vi "TEST.vi"() -> ()   [LabVIEW 2014]
uses:
  <vilib>/Instr/_visa.llb/VISA Configure Serial Port (Instr).vi
panel:
  in  "Delay":u32=1000
  in  "Network":bool
  out "Axis":string="L127M127R127"
  in  "포트":u16=50
  in  "IP":string="127.0.0.1"
  out "불리언":bool=TRUE
  out "Write":string="L127,M127,R127,;\r"
  in  "Motor R":u32(slide)=128 scale=0.0..255.0
  in  "Motor M":u32(slide)=128 scale=0.0..255.0
  in  "Motor L":u32(slide)=128 scale=0.0..255.0
  in  "정지 버튼":bool
  in  "RUN":bool
  out "WORK":i32=34
  in  "VISA resource name":refnum<visa-resource-name>="COM3"
  in  "Serial Settings":T1={"baud rate"=9600, "data bits"=8, "parity"=enum."None", "stop bits"=10, "flow control"=0} {"flow control" items=["None"=0, "XON/XOFF"=1, "RTS/CTS"=2, "DTR/DSR"=4]; "stop bits" items=["1.0"=10, "1.5"=15, "2.0"=20]; "data bits" min=5 max=8 step=1; "baud rate" items=["75"=75, "110"=110, "134"=134, "150"=150, "300"=300, "600"=600, "1200"=1200, "1800"=1800, "2400"=2400, "4800"=4800, "7200"=7200, "9600"=9600, "14400"=14400, "19200"=19200, "28800"=28800, "38400"=38400, "56000"=56000, "57600"=57600, "115200"=115200, "128000"=128000, "230400"=230400]}
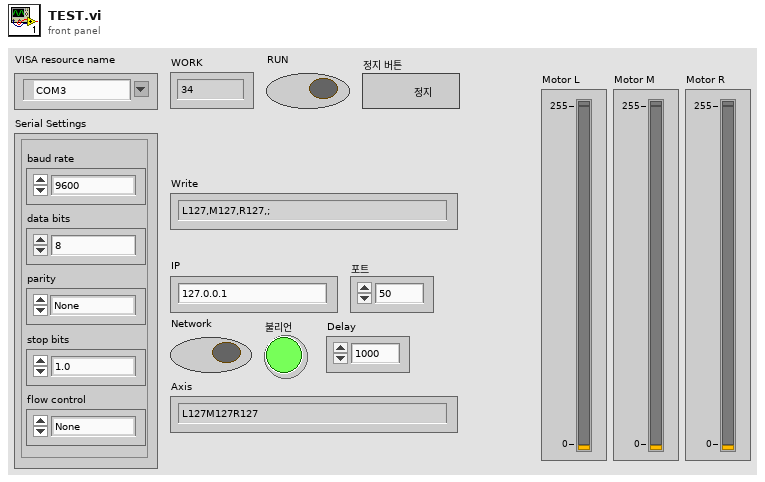
[diagram p1: front panel]
types:
  T1 = cluster{"baud rate":u32, "data bits":u16, "parity":enum16{"None", "Odd", "Even", "Mark", "Space"}, "stop bits":u16, "flow control":u16}
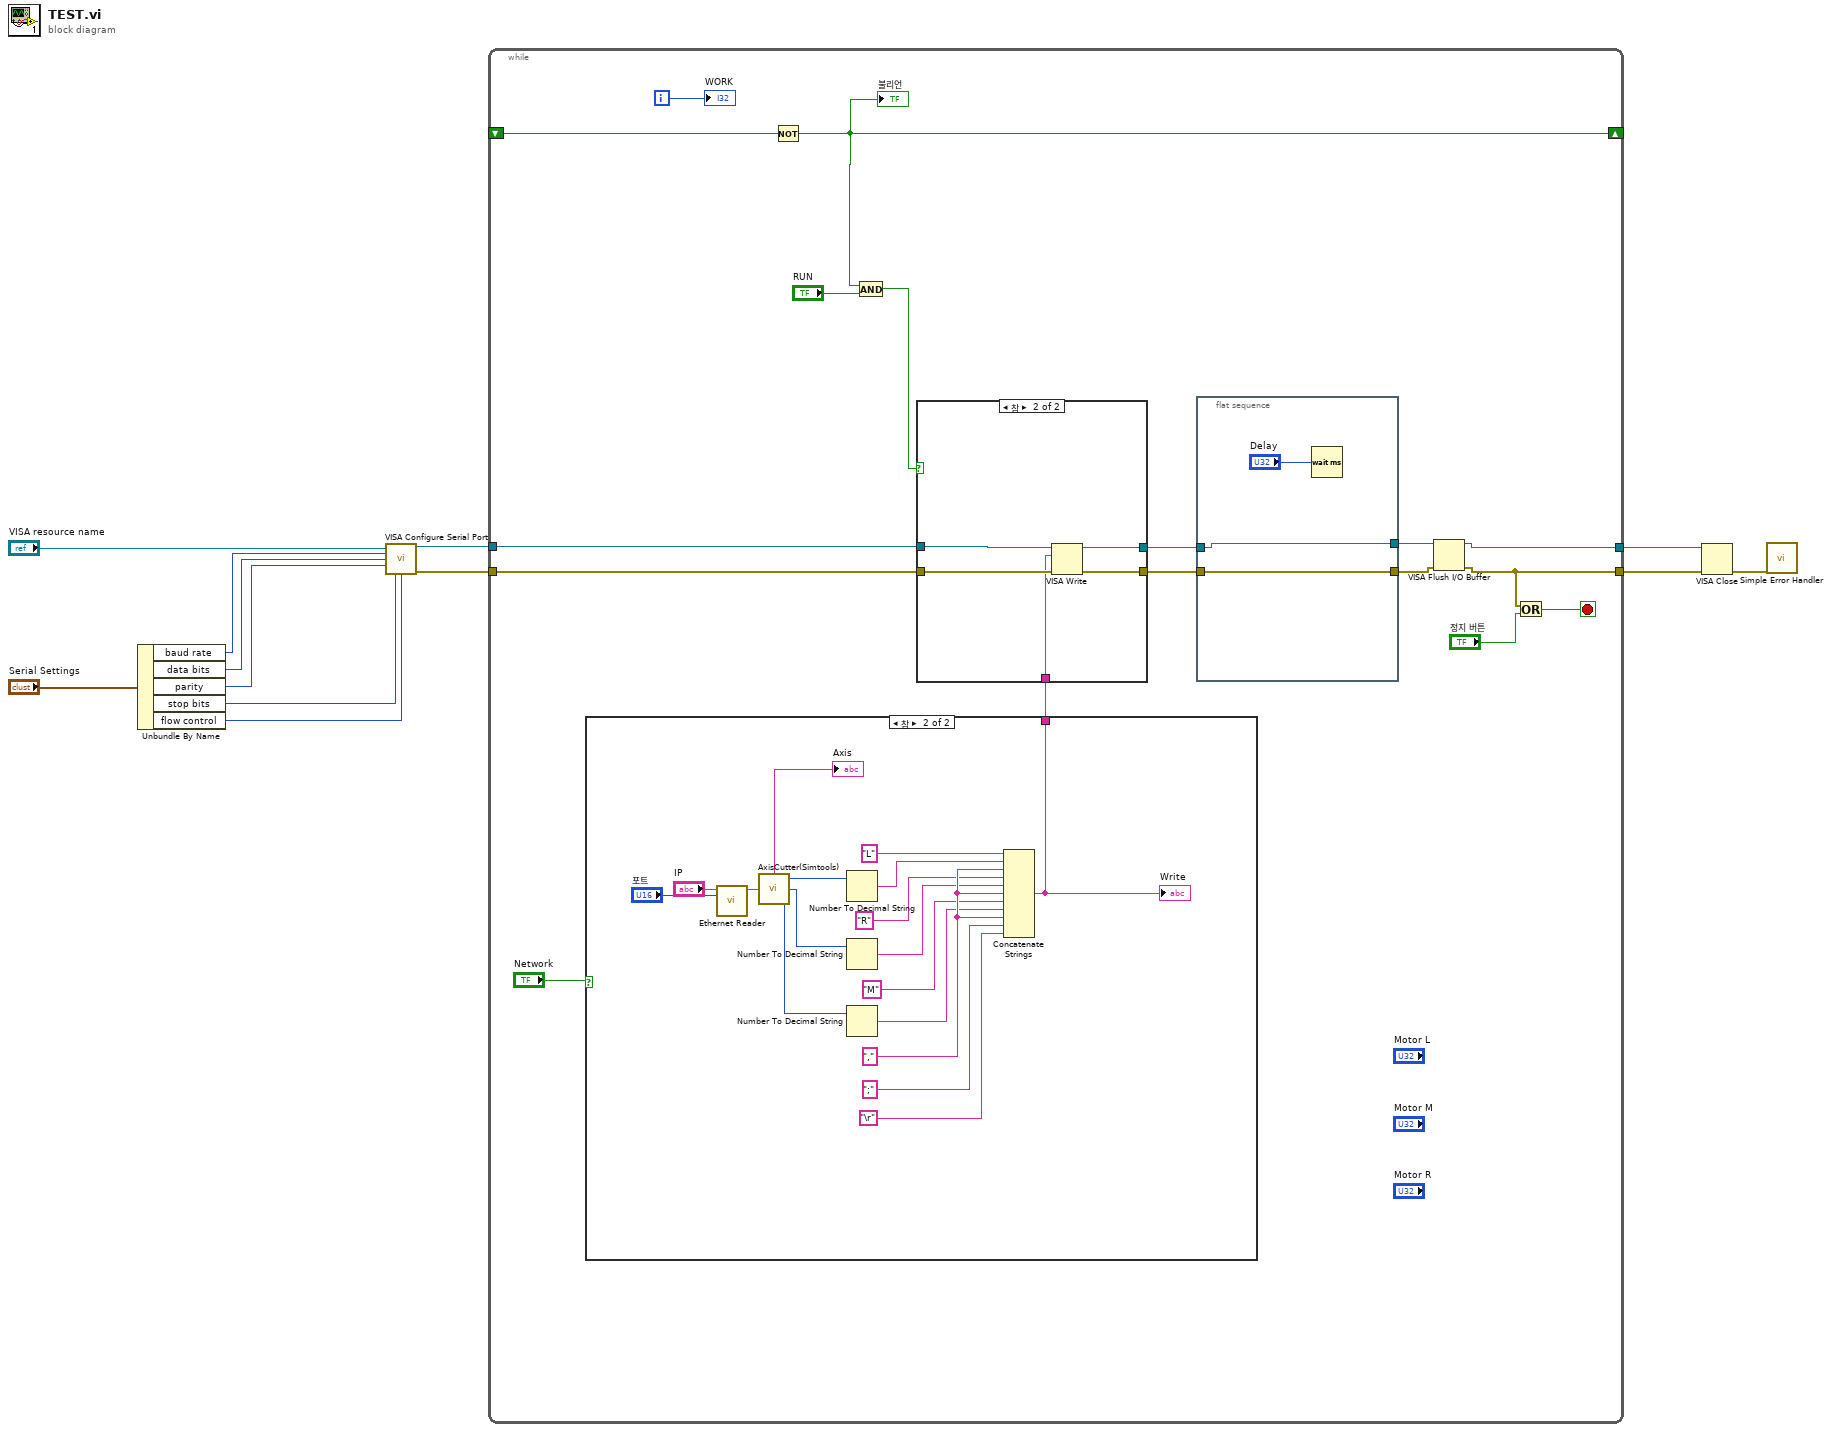
[diagram p0: block diagram]
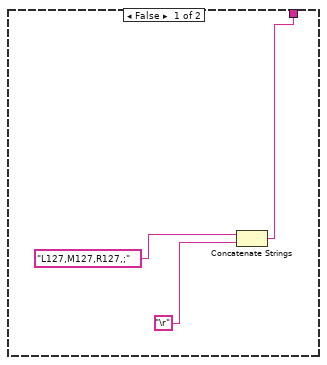
[diagram p2: hidden frame]
diagram:
  n1 = Unbundle By Name("Serial Settings") -> ("baud rate"=w5:u32, "data bits"=w4:u16, "parity"=w3:enum16{"None", "Odd", "Even", "Mark", "Space"}, "stop bits"=w2:u16, "flow control"=w1:u16)
  n2 = call-poly "VISA Configure Serial Port"("VISA resource name"="VISA resource name", "baud rate (9600)"=w5, "data bits (8)"=w4, "parity (0:none)"=w3, "stop bits (10: 1 bit)"=w2, "flow control (0:none)"=w1) -> ("VISA resource name out"=w12:refnum<visa-resource-name>, "error out"=w11:errorcluster)  [unwired: 8 in]
  n3 = while {
    tunnel: w12 -> [w29]
    tunnel: w11 -> [w28]
    tunnel: [w13] -> w9
    tunnel: [w14] -> w8
    shift-right: [w22] -> _
    shift-left: _ -> [w24]
    i -> [w27]
    stop <- w26 stop-if-true
    n4 = case shown="참" "Network" {
      tunnel: [w34 w40] -> w21
      frame False {
        n5 = Concatenate Strings("L127,M127,R127,;", "\r") -> (w34:string)
      }
      frame True {
        w50 = ","
        n6 = call "Ethernet Reader.vi"("IP"="IP", "포트"="포트") -> ("Axis"=w41:string)  [unwired: 6 in, 1 out]
        n7 = call "AxisCutter(Simtools).vi"("수신"=w41) -> ("Axis"=→"Axis":string, "L"=w39:i32, "R"=w37:i32, "M"=w36:i32)
        n8 = Number To Decimal String(number=w39) -> (decimal integer string=w51:string)  [unwired: 1 in]
        n9 = Number To Decimal String(number=w37) -> (decimal integer string=w48:string)  [unwired: 1 in]
        n10 = Number To Decimal String(number=w36) -> (decimal integer string=w46:string)  [unwired: 1 in]
        n11 = Concatenate Strings("L", w51, w50, "R", w48, w50, "M", w46, w50, ";", "\r") -> (w40:string)
        "Write" <- w40
      }
    }
    n12 = Not(x=w24) -> (.not. x?=w22:bool)
    "불리언" <- w22
    n13 = And(x=w22, y="RUN") -> (x .and. y?=w23:bool)
    n14 = case shown="참" w23 {
      tunnel: w29 -> [w54 w59]
      tunnel: w28 -> [w53 w58]
      tunnel: [w54 w56] -> w18
      tunnel: [w53 w55] -> w17
      tunnel: w21 -> [_ w57]
      frame False {
      }
      frame True {
        n15 = VISA Write(VISA resource name=w59, write buffer=w57, error in (no error)=w58) -> (VISA resource name out=w56:refnum<visa-resource-name>, error out=w55:errorcluster)  [unwired: 1 out]
      }
    }
    n16 = flat-sequence {
      tunnel: w18 -> [w31]
      tunnel: w17 -> [w30]
      tunnel: [w31] -> w16
      tunnel: [w30] -> w15
      frame #0 {
        n17 = Wait (ms)(milliseconds to wait="Delay") -> ()  [unwired: 1 out]
      }
    }
    n18 = VISA Flush I/O Buffer(VISA resource name=w16, error in (no error)=w15) -> (VISA resource name out=w13:refnum<visa-resource-name>, error out=w14:errorcluster)  [unwired: 1 in]
    n19 = Or(x=w14, y="정지 버튼") -> (x .or. y?=w26:bool)
    "WORK" <- w27
  }
  n20 = VISA Close(VISA resource name=w9, error in (no error)=w8) -> (error out=w10:errorcluster)
  n21 = call <vilib>:"Simple Error Handler.vi"("error in (no error)"=w10) -> ()  [unwired: 1 in, 8 out]
